vi "Stop Test.vi"(8 "error in (no error)":errorcluster, 10 "Test":string, 11 "Model in":refnum<class "Model.lvclass">) -> (0 "error out":errorcluster, 3 "Model out":refnum<class "Model.lvclass">)   [LabVIEW 2016, in "Model.lvclass"]
uses:
  Model.lvclass
  Model.lvclass/Model.ctl
  Common_SerialProtocols/SerialProtocol/SerialReal/SerialReal.lvclass
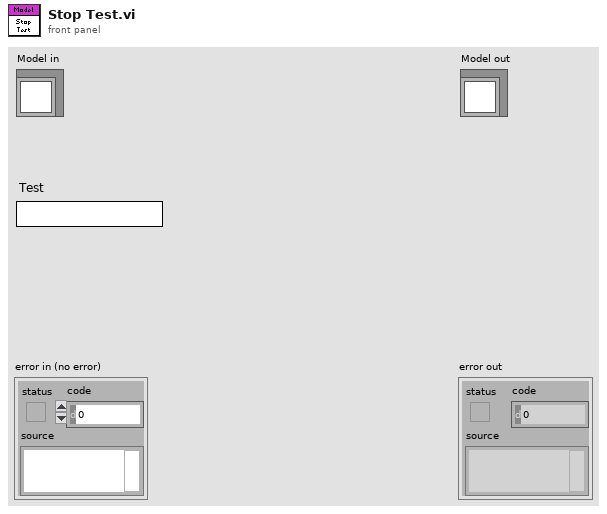
[diagram p1: front panel]
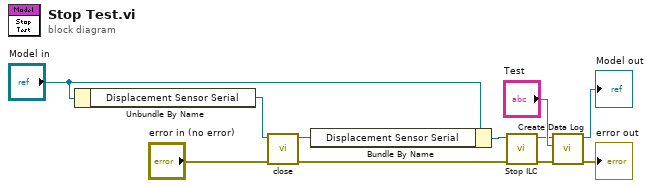
[diagram p0: block diagram]
diagram:
  n1 = Unbundle By Name("Model in") -> ("Displacement Sensor Serial"=w8:refnum<class "SerialReal.lvclass">)
  n2 = call-dynamic "close.vi"("error in (no error)"="error in (no error)", "SerialReal in"=w8) -> ("error out"=w1:errorcluster, "SerialReal out"=w6:refnum<class "SerialReal.lvclass">)  [unwired: 8 in]
  n3 = Bundle By Name(cluster="Model in", "Displacement Sensor Serial"=w6) -> (w4:refnum<class "Model.lvclass">)
  n4 = call "Stop ILC.vi"("error in (no error)"=w1, "Model in"=w4) -> ("error out"=w2:errorcluster, "Model out"=w3:refnum<class "Model.lvclass">)  [unwired: 8 in]
  n5 = call "Create Data Log.vi"("error in (no error)"=w2, "Test"="Test", "Model in"=w3) -> ("error out"=→"error out":errorcluster, "Model out"=→"Model out":refnum<class "Model.lvclass">)  [unwired: 7 in]
